vi "NiFPGA Reserve IRQs.vi"(8 "error in (no error)":errorcluster, 11 "Session In":u32) -> (0 "error out":errorcluster, 1 "Context":u32, 3 "Session Out":u32)   [LabVIEW 2010, in "FPGA Interface Wrapper.lvlib"]
doc: "IRQ contexts are single-threaded; only one thread can wait with a particular context at any given time. Clients must reserve as many contexts as the application requires. If a context is successfully reserved (the returned status is not an error), it must be unreserved later. Otherwise a memory leak will occur."
uses:
  <userlib>/_FPGA Interface Advanced Tools/FPGA Interface Wrapper/FPGA Interface Wrapper.lvlib
  NiFpga.dll
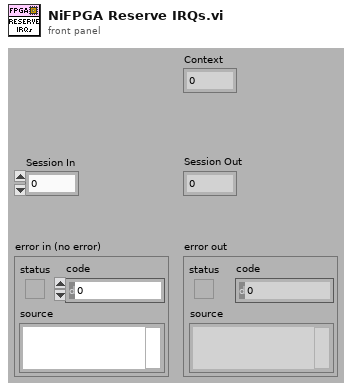
[diagram p1: front panel]
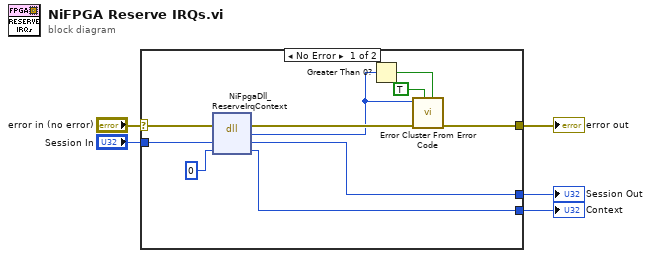
[diagram p0: block diagram]
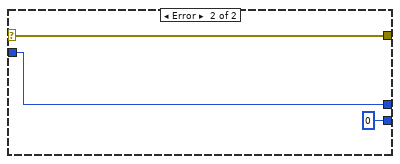
[diagram p2: hidden frame]
diagram:
  n1 = case shown="No Error" "error in (no error)" {
    selector: "error in (no error)" -> [w15 w17]
    tunnel: [w7 w17] -> w5
    tunnel: [w14 w18] -> w3
    tunnel: "Session In" -> [w13 w18]
    tunnel: [w11 u32 0 ("Context")] -> w1
    frame No Error {
      n2 = dll-call lib="NiFpga.dll" fn="NiFpgaDll_ReserveIrqContext"(error in=w15, "Session"=w13, "Context"=u32 0) -> (error out=w8:errorcluster, "Status"=w6:i32, "Session"=w14:u32, "Context"=w11:u32)  [unwired: 2 in, 1 out]
      n3 = Greater Than 0?(x=w6) -> (x > 0?=w9:bool)
      n4 = call <vilib>:"Error Cluster From Error Code.vi"("is warning? (False)"=w9, "show call chain? (False)"=TRUE, "error in (no error)"=w8, "error code (0)"=w6) -> ("error out"=w7:errorcluster)  [unwired: 5 in]
    }
    frame Error {
    }
  }
  "error out" <- w5
  "Session Out" <- w3
  "Context" <- w1
